vi "LCOS GUI v3.vi"() -> ()   [LabVIEW 2011]
uses:
  Periodic Spot Pattern Parameters.ctl
  Periodic Spot Pattern Parameters2.ctl
  LCOS State Machine States.ctl
  LCOS Pattern Display Actions.ctl
  LCOS Parent Action.ctl
  LCOS Images.ctl
  <vilib>/vision/Image Controls.llb/IMAQ Image.ctl
panel:
  in  "Enable Remote Control":bool=TRUE
  in  "Clear Error":bool
  in  "Ignore":bool
  out "Last Error":errorcluster
  in  "Loaded Pattern File:":bool
  out "File Path":path
  out "LCOS Pattern Preview":T1(plugin-control)
  in  "Buttons":T2={"Pattern"=enum."Computed", "Auto-Update LCOS"=TRUE, "Apply Correction"=FALSE, "Update LCOS"=FALSE, "Preview Pattern"=FALSE, "Auto-Preview"=TRUE}
  in  "Pattern Definition":T3={"Spot pitch (pixels)"=23.1, "Tilt Angle (deg)"=0.0, "Horizontal Offset (pixels)"=91.9, "Vertical Offset (pixels)"=14.1, "# Horizontal Spots"=8, "# Vertical Spots"=1, "Spot size (pixels)"=23.1, "Darken center spot"=FALSE, "Exact Phase Formula"=TRUE, "phase wrapping"=FALSE, "Set Focus (mm)"=32.0, "Add phase"=4.0, "phase_factor"=65.0, "Steering LW"=1.0, "Steering vmax"=0.0, "phase_overshoot"=TRUE, "Focal shift param"=0.0, "x0 focal shift"=0.0, "y0 focal shift"=0.0, "hv_steering"=TRUE, "fixed"=TRUE, "Pad"=0.0, "dark_all"=FALSE, "nospot"=FALSE, "Laser wavelength"=6.28e-07} {"Laser wavelength" min=0.0 max=500.0 format="%^#.3e"; "Pad" min=0.0 max=500.0 step=1.0 format="%#.0g"; "y0 focal shift" min=0.0 max=500.0 format="%#.3g"; "x0 focal shift" min=0.0 max=500.0 format="%#.3g"; "Focal shift param" min=0.0 max=500.0 format="%#.3g"; "Steering vmax" min=0.0 max=500.0 format="%#.3g"; "Steering LW" min=0.0 max=500.0 format="%#.3g"; "phase_factor" min=0.0 max=500.0 format="%#.3f"; "Add phase" min=0.0 max=500.0 format="%#.3f"; "Set Focus (mm)" min=0.0 max=500.0 format="%#.3g"; "Spot size (pixels)" min=1.0 format="%.2g"; "# Vertical Spots" min=1 step=1; "# Horizontal Spots" min=1 step=1; "Vertical Offset (pixels)" format="%.2f"; "Horizontal Offset (pixels)" format="%.2f"; "Tilt Angle (deg)" min=-90.0 max=90.0 format="%.2g"; "Spot pitch (pixels)" min=1.0 format="%.2g"}
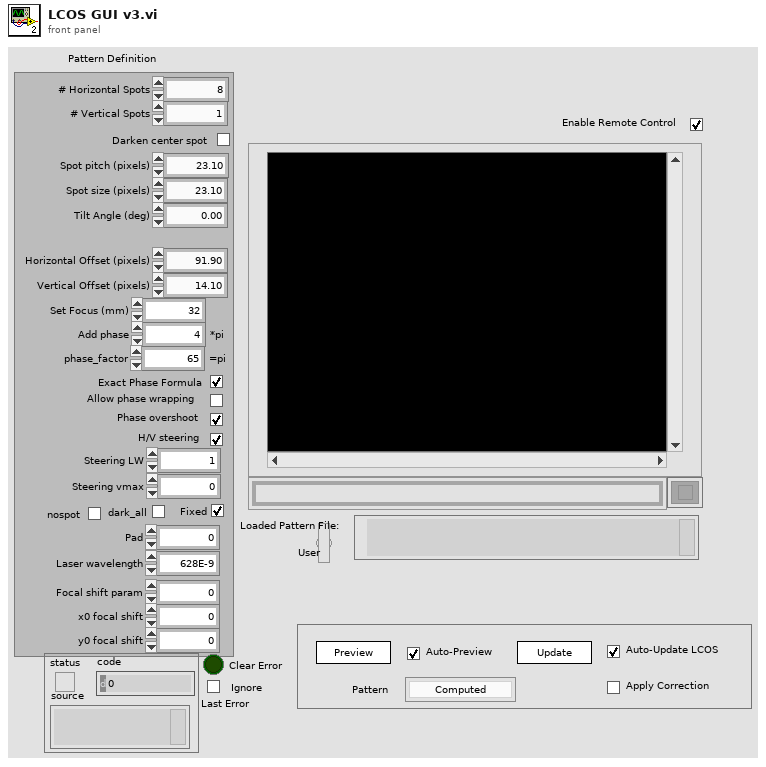
[diagram p1: front panel]
types:
  T1 = typedef "IMAQ Image.ctl" = refnum<image>
  T2 = cluster{"Pattern":enum16{"Computed", "From File", "Correction"}, "Auto-Update LCOS":bool, "Apply Correction":bool, "Update LCOS":bool, "Preview Pattern":bool, "Auto-Preview":bool}
  T3 = typedef "Periodic Spot Pattern Parameters.ctl" = cluster{"Spot pitch (pixels)":dbl, "Tilt Angle (deg)":dbl, "Horizontal Offset (pixels)":dbl, "Vertical Offset (pixels)":dbl, "# Horizontal Spots":u32, "# Vertical Spots":u32, "Spot size (pixels)":dbl, "Darken center spot":bool, "Exact Phase Formula":bool, "phase wrapping":bool, "Set Focus (mm)":T4, "Add phase":dbl, "phase_factor":dbl, "Steering LW":T4, "Steering vmax":T4, "phase_overshoot":bool, "Focal shift param":T4, "x0 focal shift":T4, "y0 focal shift":T4, "hv_steering":bool, "fixed":bool, "Pad":T4, "dark_all":bool, "nospot":bool, "Laser wavelength":dbl}
  T4 = typedef "Periodic Spot Pattern Parameters2.ctl" = dbl
  T5 = typedef "LCOS Pattern Display Actions.ctl" = enum16{"Init", "Idle", "Update", "Exit"}
  T6 = cluster{"LCOS Pattern Display Actions":T5, "Data":variant}
  T7 = typedef "LCOS State Machine States.ctl" = enum16{"Init", "Idle", "Preview Button Pushed", "Update Button Pushed", "Pattern Selection Changed", "Pattern Definition Changed", "Selected File Changed", "Load Correction Pattern", "Load Correction Pattern Step 2", "Load User Pattern", "Load User Pattern Step 2", "Compute Pattern", "Correct Pattern", "Update Preview Display", "Update LCOS Display", "Error", "Clear Error", "Exit"}
  T8 = cluster{"Spot pitch (pixels)":dbl, "Tilt Angle (deg)":dbl, "Horizontal Offset (pixels)":dbl, "Vertical Offset (pixels)":dbl, "# Horizontal Spots":u32, "# Vertical Spots":u32, "Spot size (pixels)":dbl, "Darken center spot":bool, "Exact Phase Formula":bool, "phase wrapping":bool, "Set Focus (mm)":T4, "Add phase":dbl, "phase_factor":dbl, "Steering LW":T4, "Steering vmax":T4, "phase_overshoot":bool, "Focal shift param":T4, "x0 focal shift":T4, "y0 focal shift":T4, "hv_steering":bool, "fixed":bool, "Pad":T4, "dark_all":bool, "nospot":bool, "Laser wavelength":dbl}
  T9 = typedef "LCOS Parent Action.ctl" = enum16{"Pattern Definition Changed", "Preview Button Pushed", "Update Button Pushed", "Pattern Selection Changed", "Correction Pattern Changed", "User Pattern (from File) Changed"}
  T10 = typedef "LCOS Images.ctl" = cluster{"Computed Pattern Image":T1, "User Pattern (from File) Image":T1, "Correction Pattern Image":T1, "Corrected Pattern Image":T1, "Preview Image":T1, "LCOS Displayed Image":T1}
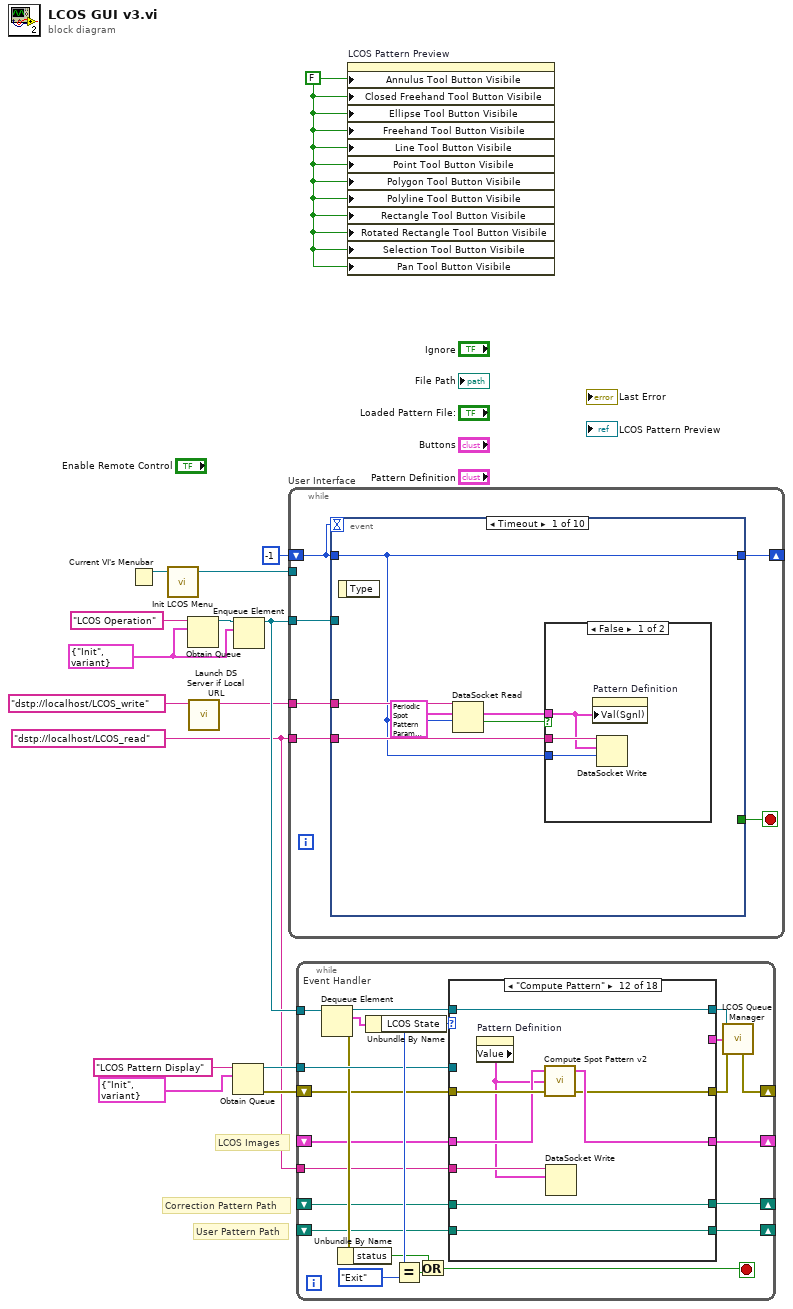
[diagram p0: block diagram]
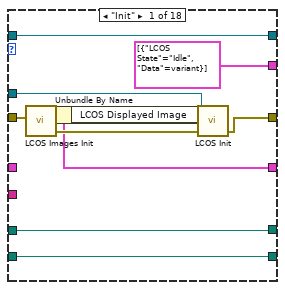
[diagram p2: hidden frame]
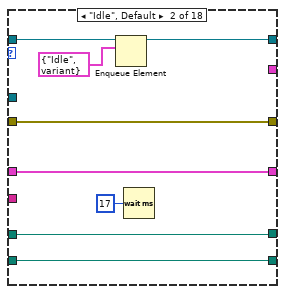
[diagram p3: hidden frame]
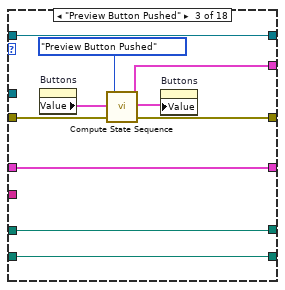
[diagram p4: hidden frame]
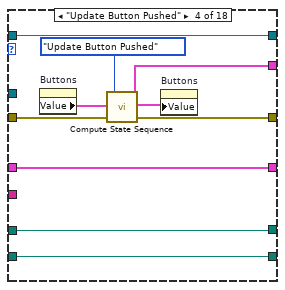
[diagram p5: hidden frame]
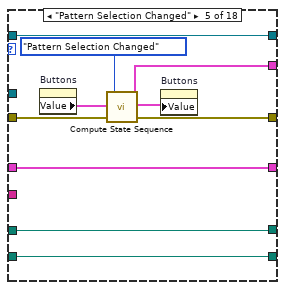
[diagram p6: hidden frame]
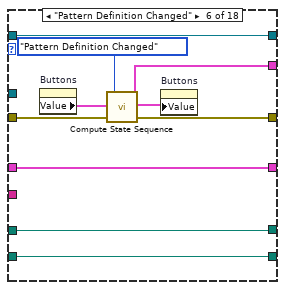
[diagram p7: hidden frame]
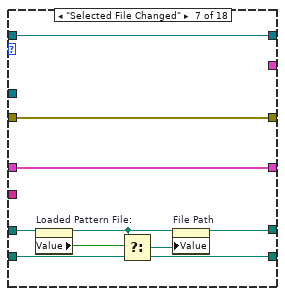
[diagram p8: hidden frame]
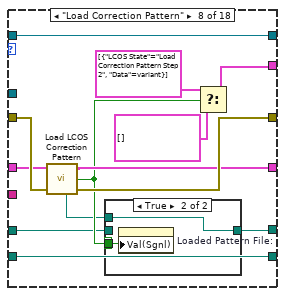
[diagram p9: hidden frame]
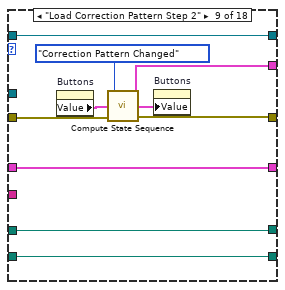
[diagram p11: hidden frame]
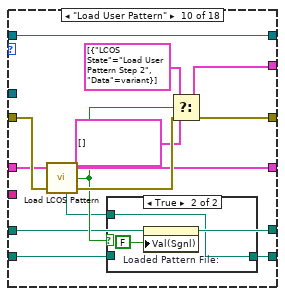
[diagram p12: hidden frame]
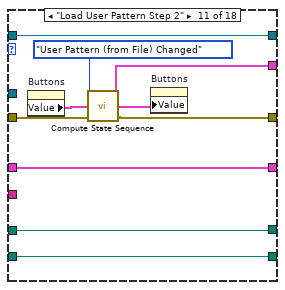
[diagram p14: hidden frame]
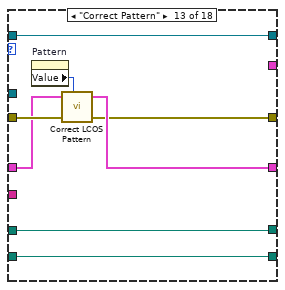
[diagram p15: hidden frame]
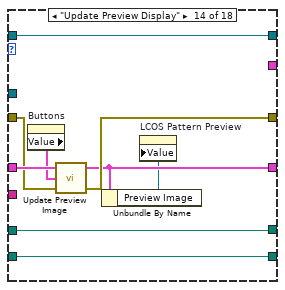
[diagram p16: hidden frame]
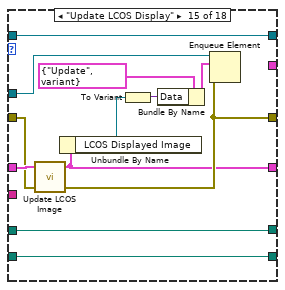
[diagram p17: hidden frame]
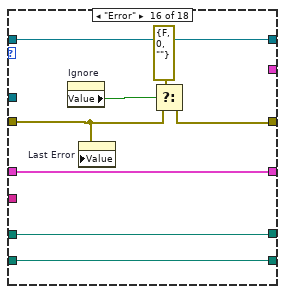
[diagram p18: hidden frame]
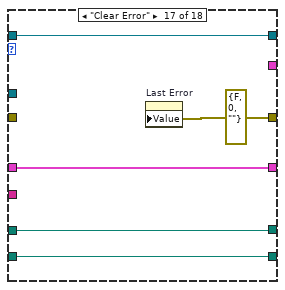
[diagram p19: hidden frame]
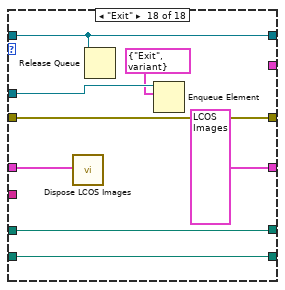
[diagram p20: hidden frame]
diagram:
  w1 = "dstp://localhost/LCOS_read" ("URL")
  w5 = FALSE ("ROI Tool Buttons Visibile:Annulus Tool Button Visibile")
  w6 = cluster{"LCOS State":T7, "Data":variant} {"LCOS State"=enum."Init", "Data"=variant}
  # "User Pattern Path"
  # "Correction Pattern Path"
  # "LCOS Images"
  n1 = Current VI's Menubar() -> (w15:refnum<k9>)
  n2 = call "Init LCOS Menu.vi"("Menu Refnum (in)"=w15) -> ("Menu Refnum (out)"=w14:refnum<k9>)  [unwired: 7 in, 1 out]
  n3 = Obtain Queue(name (unnamed)="LCOS Operation", element data type=w6) -> (queue out=w8:refnum<queue>)  [unwired: 3 in, 2 out]
  n4 = call "Launch DS Server if Local URL.vi"("URL"="dstp://localhost/LCOS_write") -> ("Duplicate URL"=w2:string)  [unwired: 5 in, 1 out]
  n5 = Obtain Queue(name (unnamed)="LCOS Pattern Display", element data type=T6 {"LCOS Pattern Display Actions"=enum."Init", "Data"=variant}) -> (queue out=w10:refnum<queue>, error out=w9:errorcluster)  [unwired: 3 in, 1 out]
  n6 = Enqueue Element(queue=w8, element=w6) -> (queue out=w7:refnum<queue>)  [unwired: 2 in, 2 out]
  n7 = while "User Interface" {
    tunnel: w14 -> [_]
    tunnel: w7 -> [w20]
    shift-right: [w19] -> _
    shift-left: -1 -> [w18]
    tunnel: w2 -> [w17]
    tunnel: w1 -> [w16]
    stop <- w21 stop-if-true
    n8 = event shown="[0] Timeout" {
      selector: _ -> [_ _ _ _ _ _ _ _ _ _]
      dyn-events: _ -> [_ _ _ _ _ _ _ _ _ _]
      timeout: w18 -> [_ _ _ _ _ _ _ _ _ _]
      tunnel: [_ _ _ _ _ _ _ _ w57 w75] -> w21
      tunnel: w20 -> [_ _ w40 w43 w46 w49 w52 w55 w58 w74]
      tunnel: [w22 w34 w38 w41 w44 w47 w50 w53 w56 w72] -> w19
      tunnel: w18 -> [w22 _ w38 w41 w44 w47 w50 w53 w56 w72]
      tunnel: w17 -> [w27 _ _ _ _ _ _ _ _ _]
      tunnel: w16 -> [w23 w31 _ _ _ _ _ _ _ _]
      event Timeout {
        n9 = event-data() -> ()  [unwired: 1 in, 1 out]
        n10 = DataSocket Read(9:w22, 10:T3 {"Spot pitch (pixels)"=0.0, "Tilt Angle (deg)"=0.0, "Horizontal Offset (pixels)"=0.0, "Vertical Offset (pixels)"=0.0, "# Horizontal Spots"=0, "# Vertical Spots"=0, "Spot size (pixels)"=0.0, "Darken center spot"=FALSE, "Exact Phase Formula"=FALSE, "phase wrapping"=FALSE, "Set Focus (mm)"=0.0, "Add phase"=0.0, "phase_factor"=0.0, "Steering LW"=0.0, "Steering vmax"=0.0, "phase_overshoot"=FALSE, "Focal shift param"=0.0, "x0 focal shift"=0.0, "y0 focal shift"=0.0, "hv_steering"=FALSE, "fixed"=FALSE, "Pad"=0.0, "dark_all"=FALSE, "nospot"=FALSE, "Laser wavelength"=0.0} ("Pattern Definition"), 11:w27) -> (1:w25:bool, 2:w24:T3)  [unwired: 2 in, 5 out]
        n11 = case shown="False" w25 {
          tunnel: w24 -> [w29 _]
          tunnel: w23 -> [w30 _]
          tunnel: w22 -> [w28 _]
          frame False {
            n12 = property on="Pattern Definition" class="Clust (strict)"("Val(Sgnl)"=w29) -> ()  [unwired: 2 in, 2 out]
            n13 = DataSocket Write(9:w28, 10:w29, 11:w30) -> ()  [unwired: 1 in, 3 out]
          }
          frame True {
          }
        }
      }
      event "Enable Remote Control": Value Change {
        n14 = event-data() -> ("NewVal"=w32:bool)  [unwired: 1 in]
        n15 = case shown="False" w32 {
          tunnel: w31 -> [_ w37]
          frame False {
          }
          frame True {
            n16 = property on="Pattern Definition" class="Clust (strict)"() -> ("Value"=w36:T8)  [unwired: 2 in, 2 out]
            n17 = DataSocket Write(10:w36, 11:w37) -> ()  [unwired: 2 in, 3 out]
          }
        }
        n18 = Select(t=1, s=w32, f=-1) -> (s? t:f=w34:i32)
      }
      event Value Change {
        n19 = event-data() -> ()  [unwired: 1 in, 1 out]
        n20 = Enqueue Element(queue=w40, element=cluster{"LCOS State":T7, "Data":variant} {"LCOS State"=enum."Pattern Definition Changed", "Data"=variant}) -> ()  [unwired: 2 in, 3 out]
      }
      event "Buttons.Preview Pattern": Value Change {
        n21 = event-data() -> ()  [unwired: 1 in, 1 out]
        n22 = Enqueue Element(queue=w43, element=cluster{"LCOS State":T7, "Data":variant} {"LCOS State"=enum."Preview Button Pushed", "Data"=variant}) -> ()  [unwired: 2 in, 3 out]
      }
      event "Buttons.Update LCOS": Value Change {
        n23 = event-data() -> ()  [unwired: 1 in, 1 out]
        n24 = Enqueue Element(queue=w46, element=cluster{"LCOS State":T7, "Data":variant} {"LCOS State"=enum."Update Button Pushed", "Data"=variant}) -> ()  [unwired: 2 in, 3 out]
      }
      event "Buttons.Pattern": Value Change {
        n25 = event-data() -> ()  [unwired: 1 in, 4 out]
        n26 = Enqueue Element(queue=w49, element=cluster{"LCOS State":T7, "Data":variant} {"LCOS State"=enum."Pattern Selection Changed", "Data"=variant}) -> ()  [unwired: 2 in, 3 out]
      }
      event "Clear Error": Value Change {
        n27 = event-data() -> ()  [unwired: 1 in, 1 out]
        n28 = Enqueue Element(queue=w52, element=cluster{"LCOS State":T7, "Data":variant} {"LCOS State"=enum."Clear Error", "Data"=variant}) -> ()  [unwired: 2 in, 3 out]
      }
      event "Loaded Pattern File:": Value Change {
        n29 = event-data() -> ()  [unwired: 1 in, 1 out]
        n30 = Enqueue Element(queue=w55, element=cluster{"LCOS State":T7, "Data":variant} {"LCOS State"=enum."Selected File Changed", "Data"=variant}) -> ()  [unwired: 2 in, 3 out]
      }
      event Menu Selection (User) {
        n31 = event-data() -> ("ItemTag"=w59:string)  [unwired: 1 in]
        n32 = case shown="\"Load Correction Pattern\"" w59 {
          tunnel: w58 -> [_ w61 w63 w67]
          tunnel: [_ _ _ w64] -> w57
          frame "-", Default {
          }
          frame "Load Correction Pattern" {
            n33 = Enqueue Element(queue=w61, element=cluster{"LCOS State":T7, "Data":variant} {"LCOS State"=enum."Load Correction Pattern", "Data"=variant}) -> ()  [unwired: 2 in, 3 out]
          }
          frame "Load User Pattern" {
            n34 = Enqueue Element(queue=w63, element=cluster{"LCOS State":T7, "Data":variant} {"LCOS State"=enum."Load User Pattern", "Data"=variant}) -> ()  [unwired: 2 in, 3 out]
          }
          frame "Quit" {
            n35 = Two Button Dialog(message="Do you want to quit?") -> (T button?=w64:bool)  [unwired: 2 in]
            n36 = case shown="True" w64 {
              tunnel: w67 -> [w68 w71]
              tunnel: [w68 w70] -> _
              tunnel: cluster{"LCOS State":T7, "Data":variant} {"LCOS State"=enum."Exit", "Data"=variant} ("element") -> [_ w69]
              frame False {
              }
              frame True {
                n37 = Enqueue Element(queue=w71, element=w69) -> (queue out=w70:refnum<queue>)  [unwired: 2 in, 2 out]
              }
            }
          }
        }
      }
      event Panel Close? {
        w75 = TRUE ("Discard?")
        n38 = event-data() -> ()  [unwired: 1 in, 1 out]
        n39 = Enqueue Element(queue=w74, element=cluster{"LCOS State":T7, "Data":variant} {"LCOS State"=enum."Exit", "Data"=variant}) -> ()  [unwired: 2 in, 3 out]
        n40 = event-data("Discard?"=w75) -> ()  [unwired: 1 in, 1 out]
      }
    }
  }
  n41 = while "Event Handler" {
    tunnel: w10 -> [w92]
    shift-right: [w86] -> _
    shift-left: w9 -> [w84]
    tunnel: w7 -> [w97]
    shift-right: [w82] -> _
    shift-left: _ -> [w83]
    shift-right: [w80] -> _
    shift-left: _ -> [w79]
    shift-right: [w78] -> _
    shift-left: _ -> [w77]
    tunnel: w1 -> [w76]
    stop <- w89 stop-if-true
    n42 = Dequeue Element(queue=w97) -> (queue out=w93:refnum<queue>, element=w91:cluster{"LCOS State":T7, "Data":variant}, error out=w90:errorcluster)  [unwired: 2 in, 1 out]
    n43 = Unbundle By Name(w90) -> ("status"=w88:bool)
    n44 = Unbundle By Name(w91) -> ("LCOS State"=w96:T7)
    n45 = Equal?(x=w96, y=LCOS_State_Machine_States."Exit") -> (x = y?=w94:bool)
    n46 = Or(x=w88, y=w94) -> (x .or. y?=w89:bool)
    n47 = case shown="\"Compute Pattern\"" w96 {
      tunnel: w93 -> [w100 w115 w122 w132 w142 w152 w162 w170 w186 w196 w212 w219 w226 w240 w248 w255 w263 w268]
      tunnel: w92 -> [w107 _ _ _ _ _ _ _ _ _ _ _ _ _ w252 _ _ w272]
      tunnel: [cluster{"LCOS State":T7, "Data":variant}[] [{"LCOS State"=enum."Idle", "Data"=variant}] ("Action Sequence") _ w119 w129 w139 w149 _ w173 w183 w198 w209 _ _ _ _ _ _ _] -> w87
      tunnel: [w106 w113 w120 w130 w140 w150 w161 w174 w184 w200 w210 w220 w227 w236 w245 w258 w265 w273] -> w85
      tunnel: w84 -> [w105 w113 w121 w131 w141 w151 w161 w175 w185 w201 w211 w223 w230 w237 w246 w256 _ w273]
      tunnel: w83 -> [_ w111 w124 w134 w144 w154 w160 w169 w181 w195 w207 w222 w229 w239 w247 w260 w264 w270]
      tunnel: [w102 w111 w124 w134 w144 w154 w160 w168 w181 w194 w207 w221 w228 w235 w244 w260 w264 T10 {"Computed Pattern Image"=refnum, "User Pattern (from File) Image"=refnum, "Correction Pattern Image"=refnum, "Corrected Pattern Image"=refnum, "Preview Image"=refnum, "LCOS Displayed Image"=refnum} ("Images")] -> w82
      tunnel: [w100 w110 w122 w132 w142 w152 w162 w170 w186 w196 w212 w219 w226 w240 w248 w255 w263 w268] -> w81
      tunnel: [w99 w109 w117 w127 w137 w147 w157 w165 w180 w189 w206 w218 w225 w233 w242 w254 w262 w267] -> w80
      tunnel: w79 -> [w99 w109 w117 w127 w137 w147 w157 w166 w180 w189 w206 w218 w225 w233 w242 w254 w262 w267]
      tunnel: [w98 w108 w116 w126 w136 w146 w158 w163 w179 w191 w205 w217 w224 w232 w241 w253 w261 w266] -> w78
      tunnel: w77 -> [w98 w108 w116 w126 w136 w146 w158 w163 w179 w190 w205 w217 w224 w232 w241 w253 w261 w266]
      tunnel: w76 -> [_ _ _ _ _ _ _ _ _ _ _ w216 _ _ _ _ _ _]
      frame "Init" {
        n48 = call "LCOS Images Init.vi"("error in (no error)"=w105) -> ("Images"=w102:T10, "error out"=w104:errorcluster)  [unwired: 7 in]
        n49 = Unbundle By Name(w102) -> ("LCOS Displayed Image"=w103:T1)
        n50 = call "LCOS Init.vi"("LCOS Display Queue"=w107, "LCOS Displayed Image"=w103, "error in (no error)"=w104) -> ("error out"=w106:errorcluster)  [unwired: 6 in]
      }
      frame "Idle", Default {
        n51 = Enqueue Element(queue=w115, element=cluster{"LCOS State":T7, "Data":variant} {"LCOS State"=enum."Idle", "Data"=variant}) -> (queue out=w110:refnum<queue>)  [unwired: 2 in, 2 out]
        n52 = Wait (ms)(milliseconds to wait=u32 17) -> ()  [unwired: 1 out]
      }
      frame "Preview Button Pushed" {
        n53 = property on="Buttons" class="Clust (strict)"() -> ("Value"=w125:T2)  [unwired: 2 in, 2 out]
        n54 = call "Compute State Sequence.vi"("Parent Action"=LCOS_Parent_Action."Preview Button Pushed" ("Previous Event"), "Buttons (in)"=w125, "error in (no error)"=w121) -> ("Action Sequence"=w119:cluster{"LCOS State":T7, "Data":variant}[], "Buttons (out)"=w118:T2, "error out"=w120:errorcluster)  [unwired: 4 in]
        n55 = property on="Buttons" class="Clust (strict)"("Value"=w118) -> ()  [unwired: 2 in, 2 out]
      }
      frame "Update Button Pushed" {
        n56 = property on="Buttons" class="Clust (strict)"() -> ("Value"=w135:T2)  [unwired: 2 in, 2 out]
        n57 = call "Compute State Sequence.vi"("Parent Action"=LCOS_Parent_Action."Update Button Pushed" ("Previous Event"), "Buttons (in)"=w135, "error in (no error)"=w131) -> ("Action Sequence"=w129:cluster{"LCOS State":T7, "Data":variant}[], "Buttons (out)"=w128:T2, "error out"=w130:errorcluster)  [unwired: 4 in]
        n58 = property on="Buttons" class="Clust (strict)"("Value"=w128) -> ()  [unwired: 2 in, 2 out]
      }
      frame "Pattern Selection Changed" {
        n59 = property on="Buttons" class="Clust (strict)"() -> ("Value"=w145:T2)  [unwired: 2 in, 2 out]
        n60 = call "Compute State Sequence.vi"("Parent Action"=LCOS_Parent_Action."Pattern Selection Changed" ("Previous Event"), "Buttons (in)"=w145, "error in (no error)"=w141) -> ("Action Sequence"=w139:cluster{"LCOS State":T7, "Data":variant}[], "Buttons (out)"=w138:T2, "error out"=w140:errorcluster)  [unwired: 4 in]
        n61 = property on="Buttons" class="Clust (strict)"("Value"=w138) -> ()  [unwired: 2 in, 2 out]
      }
      frame "Pattern Definition Changed" {
        n62 = property on="Buttons" class="Clust (strict)"() -> ("Value"=w155:T2)  [unwired: 2 in, 2 out]
        n63 = call "Compute State Sequence.vi"("Parent Action"=LCOS_Parent_Action."Pattern Definition Changed" ("Previous Event"), "Buttons (in)"=w155, "error in (no error)"=w151) -> ("Action Sequence"=w149:cluster{"LCOS State":T7, "Data":variant}[], "Buttons (out)"=w148:T2, "error out"=w150:errorcluster)  [unwired: 4 in]
        n64 = property on="Buttons" class="Clust (strict)"("Value"=w148) -> ()  [unwired: 2 in, 2 out]
      }
      frame "Selected File Changed" {
        n65 = property on="Loaded Pattern File:" class="Bool (strict)"() -> ("Value"=w159:bool)  [unwired: 2 in, 2 out]
        n66 = Select(t=w157, s=w159, f=w158) -> (s? t:f=w156:path)
        n67 = property on="File Path" class="Path"("Value"=w156) -> ()  [unwired: 2 in, 2 out]
      }
      frame "Load Correction Pattern" {
        n68 = call "Load LCOS Correction Pattern.vi"("Images Dest"=w169, "error in"=w175) -> ("Images Out"=w168:T10, "Correct File Type"=w167:bool, "Path"=w164:path, "error out"=w174:errorcluster)  [unwired: 3 in, 1 out]
        n69 = case shown="True" w167 {
          tunnel: w167 -> [_ w178]
          tunnel: w166 -> [w176 _]
          tunnel: [w176 w177] -> w165
          tunnel: w164 -> [_ w177]
          frame False {
          }
          frame True {
            n70 = property on="Loaded Pattern File:" class="Bool (strict)"("Val(Sgnl)"=w178) -> ()  [unwired: 2 in, 2 out]
          }
        }
        n71 = Select(t=cluster{"LCOS State":T7, "Data":variant}[] [{"LCOS State"=enum."Load Correction Pattern Step 2", "Data"=variant}], s=w167, f=cluster{"LCOS State":T7, "Data":variant}[] []) -> (s? t:f=w173:cluster{"LCOS State":T7, "Data":variant}[])
      }
      frame "Load Correction Pattern Step 2" {
        n72 = property on="Buttons" class="Clust (strict)"() -> ("Value"=w188:T2)  [unwired: 2 in, 2 out]
        n73 = call "Compute State Sequence.vi"("Parent Action"=LCOS_Parent_Action."Correction Pattern Changed" ("Previous Event"), "Buttons (in)"=w188, "error in (no error)"=w185) -> ("Action Sequence"=w183:cluster{"LCOS State":T7, "Data":variant}[], "Buttons (out)"=w182:T2, "error out"=w184:errorcluster)  [unwired: 4 in]
        n74 = property on="Buttons" class="Clust (strict)"("Value"=w182) -> ()  [unwired: 2 in, 2 out]
      }
      frame "Load User Pattern" {
        n75 = call "Load LCOS Pattern.vi"("Images Dest"=w195, "error in"=w201) -> ("Images Out"=w194:T10, "Correct File Type"=w193:bool, "Path"=w192:path, "error out"=w200:errorcluster)  [unwired: 3 in, 1 out]
        n76 = case shown="True" w193 {
          tunnel: w190 -> [w202 _]
          tunnel: [w202 w204] -> w191
          tunnel: w192 -> [_ w204]
          frame False {
          }
          frame True {
            n77 = property on="Loaded Pattern File:" class="Bool (strict)"("Val(Sgnl)"=FALSE ("Value (Signaling)")) -> ()  [unwired: 2 in, 2 out]
          }
        }
        n78 = Select(t=cluster{"LCOS State":T7, "Data":variant}[] [{"LCOS State"=enum."Load User Pattern Step 2", "Data"=variant}], s=w193, f=cluster{"LCOS State":T7, "Data":variant}[] []) -> (s? t:f=w198:cluster{"LCOS State":T7, "Data":variant}[])
      }
      frame "Load User Pattern Step 2" {
        n79 = property on="Buttons" class="Clust (strict)"() -> ("Value"=w214:T2)  [unwired: 2 in, 2 out]
        n80 = call "Compute State Sequence.vi"("Parent Action"=LCOS_Parent_Action."User Pattern (from File) Changed" ("Previous Event"), "Buttons (in)"=w214, "error in (no error)"=w211) -> ("Action Sequence"=w209:cluster{"LCOS State":T7, "Data":variant}[], "Buttons (out)"=w208:T2, "error out"=w210:errorcluster)  [unwired: 4 in]
        n81 = property on="Buttons" class="Clust (strict)"("Value"=w208) -> ()  [unwired: 2 in, 2 out]
      }
      frame "Compute Pattern" {
        n82 = property on="Pattern Definition" class="Clust (strict)"() -> ("Value"=w215:T8)  [unwired: 2 in, 2 out]
        n83 = call "Compute Spot Pattern v2.vi"("Images Dest"=w222, "Pattern Definition"=w215, "error in"=w223) -> ("Images Out"=w221:T10, "error out"=w220:errorcluster)  [unwired: 3 in, 2 out]
        n84 = DataSocket Write(10:w215, 11:w216) -> ()  [unwired: 2 in, 3 out]
      }
      frame "Correct Pattern" {
        n85 = property on="Pattern" class="Enum (strict)"() -> ("Value"=w231:enum16{"Computed", "From File", "Correction"})  [unwired: 2 in, 2 out]
        n86 = call "Correct LCOS Pattern.vi"("Images Dest"=w229, "Pattern"=w231, "error in"=w230) -> ("Images Out"=w228:T10, "error out"=w227:errorcluster)  [unwired: 5 in]
      }
      frame "Update Preview Display" {
        n87 = property on="Buttons" class="Clust (strict)"() -> ("Value"=w238:T2)  [unwired: 2 in, 2 out]
        n88 = call "Update Preview Image.vi"("Images (Dest)"=w239, "Buttons"=w238, "error in"=w237) -> ("Images (Out)"=w235:T10, "error out"=w236:errorcluster)  [unwired: 5 in]
        n89 = Unbundle By Name(w235) -> ("Preview Image"=w234:T1)
        n90 = property on="LCOS Pattern Preview" class="ImageControl"("Value"=w234) -> ()  [unwired: 2 in, 2 out]
      }
      frame "Update LCOS Display" {
        n91 = call "Update LCOS Image.vi"("Images (Dest)"=w247, "error in"=w246) -> ("Images (Out)"=w244:T10, "error out"=w245:errorcluster)  [unwired: 6 in]
        n92 = Unbundle By Name(w244) -> ("LCOS Displayed Image"=w243:T1)
        n93 = To Variant(anything=w243) -> (Variant=w249:variant)
        n94 = Bundle By Name(cluster=T6 {"LCOS Pattern Display Actions"=enum."Update", "Data"=variant}, "Data"=w249) -> (w250:T6)
        n95 = Enqueue Element(queue=w252, element=w250, error in (no error)=w245) -> ()  [unwired: 1 in, 3 out]
      }
      frame "Error" {
        n96 = property on="Ignore" class="Bool (strict)"() -> ("Value"=w259:bool)  [unwired: 2 in, 2 out]
        n97 = property on="Last Error" class="Clust (strict)"("Value"=w256) -> ()  [unwired: 2 in, 2 out]
        n98 = Select(t=errorcluster {"status"=FALSE, "code"=0, "source"=""}, s=w259, f=w256) -> (s? t:f=w258:errorcluster)
      }
      frame "Clear Error" {
        w265 = errorcluster {"status"=FALSE, "code"=0, "source"=""} ("error out")
        n99 = property on="Last Error" class="Clust (strict)"("Value"=w265) -> ()  [unwired: 2 in, 2 out]
      }
      frame "Exit" {
        n100 = call "Dispose LCOS Images.vi"("Images"=w270) -> ()
        n101 = Release Queue(queue=w268) -> ()  [unwired: 2 in, 3 out]
        n102 = Enqueue Element(queue=w272, element=T6 {"LCOS Pattern Display Actions"=enum."Exit", "Data"=variant}) -> ()  [unwired: 2 in, 3 out]
      }
    }
    n103 = call "LCOS Queue Manager.vi"("Queue"=w81, "Queue States"=w87, "error in (no error)"=w85) -> ("error out"=w86:errorcluster)  [unwired: 6 in]
  }
  n104 = property on="LCOS Pattern Preview" class="ImageControl"("Annulus Tool Button Visibile"=w5, "Closed Freehand Tool Button Visibile"=w5, "Ellipse Tool Button Visibile"=w5, "Freehand Tool Button Visibile"=w5, "Line Tool Button Visibile"=w5, "Point Tool Button Visibile"=w5, "Polygon Tool Button Visibile"=w5, "Polyline Tool Button Visibile"=w5, "Rectangle Tool Button Visibile"=w5, "Rotated Rectangle Tool Button Visibile"=w5, "Selection Tool Button Visibile"=w5, "Pan Tool Button Visibile"=w5) -> ()  [unwired: 2 in, 2 out]
